vi "nanocal -- nuclear schottky fit V8.vi"() -> ()   [LabVIEW 2021] (continued)
\"στN\" -> 0.000000000000   ,  \"τ11 \" -> 0.000000000000   ,  \"τ12\" -> 0.000000000000   ,  \"τ22\" -> 0.000000000000   ,  \"τN1\" -> 0.000000000000   ,  \"τN2\" -> 0.000000000000   ,  \"σηlogτ1 \" -> 0.000000000000   ,  \"σηlogτS\" -> 0.000000000000   ,  \"σηlogτN\" -> 0.000000000000   ,  \"σlogτ1\" -> 0.000000000000   ,  \"σlogτS\" -> 0.000000000000   ,  \"σlogτN\" -> 0.000000000000   ,  \"σητ1\" -> 0.000000000000   ,  \"σητS \" -> 0.000000000000   ,  \"σητN\" -> 0.000000000000    |>   , \r\"IDS0217_210310_RAW_cal__ref_\" ->   <|    \"ζ\" -> 0.121305227705   ,  \"τ1\" -> 0.032098202143   ,  \"τS\" -> 0.011865067519   ,  \"τN\" -> 0.005878702730   ,  \"τC\" -> 0.002147559783   ,  \"κ0\" -> 0.000000001032   ,  \"mm1\" -> 0.000202614262   ,  \"mm2\" -> 0.011552455211   ,  \"mm3\" -> 0.042386874792   ,  \"T\" -> 0.197000000000   ,  \"B\" -> 0.000000000000   ,  \"θ\" -> 0.000000000000   ,  \"Reoff\" -> 0.000000000000   ,  \"Imoff\" -> 0.000000000000   ,  \"στ1\" -> 0.000000000000   ,  \"στS\" -> 0.000000000000   ,  \"στN\" -> 0.000000000000   ,  \"τ11 \" -> 0.000000000000   ,  \"τ12\" -> 0.000000000000   ,  \"τ22\" -> 0.000000000000   ,  \"τN1\" -> 0.000000000000   ,  \"τN2\" -> 0.000000000000   ,  \"σηlogτ1 \" -> 0.000000000000   ,  \"σηlogτS\" -> 0.000000000000   ,  \"σηlogτN\" -> 0.000000000000   ,  \"σlogτ1\" -> 0.000000000000   ,  \"σlogτS\" -> 0.000000000000   ,  \"σlogτN\" -> 0.000000000000   ,  \"σητ1\" -> 0.000000000000   ,  \"σητS \" -> 0.000000000000   ,  \"σητN\" -> 0.000000000000    |>   , \r\"IDS0217_210310_RAW_cal__sam_\" ->   <|    \"ζ\" -> 0.101804363109   ,  \"τ1\" -> 0.031947692776   ,  \"τS\" -> 0.014125667853   ,  \"τN\" -> 0.006009042128   ,  \"τC\" -> 0.002323789932   ,  \"κ0\" -> 0.000000001168   ,  \"mm1\" -> 0.000188754224   ,  \"mm2\" -> 0.013103876414   ,  \"mm3\" -> 0.043163363377   ,  \"T\" -> 0.197000000000   ,  \"B\" -> 0.000000000000   ,  \"θ\" -> 0.000000000000   ,  \"Reoff\" -> 0.000000000000   ,  \"Imoff\" -> 0.000000000000   ,  \"στ1\" -> 0.000000000000   ,  \"στS\" -> 0.000000000000   ,  \"στN\" -> 0.000000000000   ,  \"τ11 \" -> 0.000000000000   ,  \"τ12\" -> 0.000000000000   ,  \"τ22\" -> 0.000000000000   ,  \"τN1\" -> 0.000000000000   ,  \"τN2\" -> 0.000000000000   ,  \"σηlogτ1 \" -> 0.000000000000   ,  \"σηlogτS\" -> 0.000000000000   ,  \"σηlogτN\" -> 0.000000000000   ,  \"σlogτ1\" -> 0.000000000000   ,  \"σlogτS\" -> 0.000000000000   ,  \"σlogτN\" -> 0.000000000000   ,  \"σητ1\" -> 0.000000000000   ,  \"σητS \" -> 0.000000000000   ,  \"σητN\" -> 0.000000000000    |>   , \r\"IDS0218_210310_RAW_cal__ref_\" ->   <|    \"ζ\" -> 0.000000000000   ,  \"τ1\" -> 0.000000000000   ,  \"τS\" -> 0.000000000000   ,  \"τN\" -> 0.000000000000   ,  \"τC\" -> 0.000000000000   ,  \"κ0\" -> 0.000000000000   ,  \"mm1\" -> 0.000000000000   ,  \"mm2\" -> 0.000000000000   ,  \"mm3\" -> 0.000000000000   ,  \"T\" -> 1.550000000000   ,  \"B\" -> 0.000000000000   ,  \"θ\" -> 0.000000000000   ,  \"Reoff\" -> 0.000000000000   ,  \"Imoff\" -> 0.000000000000   ,  \"στ1\" -> 0.000000000000   ,  \"στS\" -> 0.000000000000   ,  \"στN\" -> 0.000000000000   ,  \"τ11 \" -> 0.000000000000   ,  \"τ12\" -> 0.000000000000   ,  \"τ22\" -> 0.000000000000   ,  \"τN1\" -> 0.000000000000   ,  \"τN2\" -> 0.000000000000   ,  \"σηlogτ1 \" -> 0.000000000000   ,  \"σηlogτS\" -> 0.000000000000   ,  \"σηlogτN\" -> 0.000000000000   ,  \"σlogτ1\" -> 0.000000000000   ,  \"σlogτS\" -> 0.000000000000   ,  \"σlogτN\" -> 0.000000000000   ,  \"σητ1\" -> 0.000000000000   ,  \"σητS \" -> 0.000000000000   ,  \"σητN\" -> 0.000000000000    |>   , \r\"IDS0218_210310_RAW_cal__sam_\" ->   <|    \"ζ\" -> 0.008537038929   ,  \"τ1\" -> 0.006154643814   ,  \"τS\" -> 0.040521205127   ,  \"τN\" -> 0.000711776675   ,  \"τC\" -> 0.001925410383   ,  \"κ0\" -> 0.000000011800   ,  \"mm1\" -> 0.000015570479   ,  \"mm2\" -> 0.006036709260   ,  \"mm3\" -> 0.043612763831   ,  \"T\" -> 1.550000000000   ,  \"B\" -> 0.000000000000   ,  \"θ\" -> 0.000000000000   ,  \"Reoff\" -> -420408.163265306153   ,  \"Imoff\" -> 0.000000000000   ,  \"στ1\" -> 0.000216261088   ,  \"στS\" -> 0.000541561495   ,  \"στN\" -> 0.000022390164   ,  \"τ11 \" -> 0.000000000000   ,  \"τ12\" -> 0.000000000000   ,  \"τ22\" -> 0.000000000000   ,  \"τN1\" -> 0.000000000000   ,  \"τN2\" -> 0.000000000000   ,  \"σηlogτ1 \" -> 0.000000000000   ,  \"σηlogτS\" -> 0.000000000000   ,  \"σηlogτN\" -> 0.000000000000   ,  \"σlogτ1\" -> 0.000000000000   ,  \"σlogτS\" -> 0.000000000000   ,  \"σlogτN\" -> 0.000000000000   ,  \"σητ1\" -> 0.000000000000   ,  \"σητS \" -> 0.000000000000   ,  \"σητN\" -> 0.000000000000    |>   , \r\"IDS0219_210310_RAW_cal__ref_\" ->   <|    \"ζ\" -> 0.000000000000   ,  \"τ1\" -> 0.000000000000   ,  \"τS\" -> 0.000000000000   ,  \"τN\" -> 0.000000000000   ,  \"τC\" -> 0.000000000000   ,  \"κ0\" -> 0.000000000000   ,  \"mm1\" -> 0.000000000000   ,  \"mm2\" -> 0.000000000000   ,  \"mm3\" -> 0.000000000000   ,  \"T\" -> 1.000000000000   ,  \"B\" -> 0.000000000000   ,  \"θ\" -> 0.000000000000   ,  \"Reoff\" -> 0.000000000000   ,  \"Imoff\" -> 0.000000000000   ,  \"στ1\" -> 0.000000000000   ,  \"στS\" -> 0.000000000000   ,  \"στN\" -> 0.000000000000   ,  \"τ11 \" -> 0.000000000000   ,  \"τ12\" -> 0.000000000000   ,  \"τ22\" -> 0.000000000000   ,  \"τN1\" -> 0.000000000000   ,  \"τN2\" -> 0.000000000000   ,  \"σηlogτ1 \" -> 0.000000000000   ,  \"σηlogτS\" -> 0.000000000000   ,  \"σηlogτN\" -> 0.000000000000   ,  \"σlogτ1\" -> 0.000000000000   ,  \"σlogτS\" -> 0.000000000000   ,  \"σlogτN\" -> 0.000000000000   ,  \"σητ1\" -> 0.000000000000   ,  \"σητS \" -> 0.000000000000   ,  \"σητN\" -> 0.000000000000    |>   , \r\"IDS0219_210310_RAW_cal__sam_\" ->   <|    \"ζ\" -> 0.000000000000   ,  \"τ1\" -> 0.000000000000   ,  \"τS\" -> 0.000000000000   ,  \"τN\" -> 0.000000000000   ,  \"τC\" -> 0.000000000000   ,  \"κ0\" -> 0.000000000000   ,  \"mm1\" -> 0.000000000000   ,  \"mm2\" -> 0.000000000000   ,  \"mm3\" -> 0.000000000000   ,  \"T\" -> 1.000000000000   ,  \"B\" -> 0.000000000000   ,  \"θ\" -> 0.000000000000   ,  \"Reoff\" -> 0.000000000000   ,  \"Imoff\" -> 0.000000000000   ,  \"στ1\" -> 0.000000000000   ,  \"στS\" -> 0.000000000000   ,  \"στN\" -> 0.000000000000   ,  \"τ11 \" -> 0.000000000000   ,  \"τ12\" -> 0.000000000000   ,  \"τ22\" -> 0.000000000000   ,  \"τN1\" -> 0.000000000000   ,  \"τN2\" -> 0.000000000000   ,  \"σηlogτ1 \" -> 0.000000000000   ,  \"σηlogτS\" -> 0.000000000000   ,  \"σηlogτN\" -> 0.000000000000   ,  \"σlogτ1\" -> 0.000000000000   ,  \"σlogτS\" -> 0.000000000000   ,  \"σlogτN\" -> 0.000000000000   ,  \"σητ1\" -> 0.000000000000   ,  \"σητS \" -> 0.000000000000   ,  \"σητN\" -> 0.000000000000    |>   , \r\"IDS0220_210310_RAW_cal__ref_\" ->   <|    \"ζ\" -> 0.000000000000   ,  \"τ1\" -> 0.000000000000   ,  \"τS\" -> 0.000000000000   ,  \"τN\" -> 0.000000000000   ,  \"τC\" -> 0.000000000000   ,  \"κ0\" -> 0.000000000000   ,  \"mm1\" -> 0.000000000000   ,  \"mm2\" -> 0.000000000000   ,  \"mm3\" -> 0.000000000000   ,  \"T\" -> 0.677000000000   ,  \"B\" -> 0.000000000000   ,  \"θ\" -> 0.000000000000   ,  \"Reoff\" -> 0.000000000000   ,  \"Imoff\" -> 0.000000000000   ,  \"στ1\" -> 0.000000000000   ,  \"στS\" -> 0.000000000000   ,  \"στN\" -> 0.000000000000   ,  \"τ11 \" -> 0.000000000000   ,  \"τ12\" -> 0.000000000000   ,  \"τ22\" -> 0.000000000000   ,  \"τN1\" -> 0.000000000000   ,  \"τN2\" -> 0.000000000000   ,  \"σηlogτ1 \" -> 0.000000000000   ,  \"σηlogτS\" -> 0.000000000000   ,  \"σηlogτN\" -> 0.000000000000   ,  \"σlogτ1\" -> 0.000000000000   ,  \"σlogτS\" -> 0.000000000000   ,  \"σlogτN\" -> 0.000000000000   ,  \"σητ1\" -> 0.000000000000   ,  \"σητS \" -> 0.000000000000   ,  \"σητN\" -> 0.000000000000    |>   , \r\"IDS0220_210310_RAW_cal__sam_\" ->   <|    \"ζ\" -> 0.000000000000   ,  \"τ1\" -> 0.000000000000   ,  \"τS\" -> 0.000000000000   ,  \"τN\" -> 0.000000000000   ,  \"τC\" -> 0.000000000000   ,  \"κ0\" -> 0.000000000000   ,  \"mm1\" -> 0.000000000000   ,  \"mm2\" -> 0.000000000000   ,  \"mm3\" -> 0.000000000000   ,  \"T\" -> 0.677000000000   ,  \"B\" -> 0.000000000000   ,  \"θ\" -> 0.000000000000   ,  \"Reoff\" -> 0.000000000000   ,  \"Imoff\" -> 0.000000000000   ,  \"στ1\" -> 0.000000000000   ,  \"στS\" -> 0.000000000000   ,  \"στN\" -> 0.000000000000   ,  \"τ11 \" -> 0.000000000000   ,  \"τ12\" -> 0.000000000000   ,  \"τ22\" -> 0.000000000000   ,  \"τN1\" -> 0.000000000000   ,  \"τN2\" -> 0.000000000000   ,  \"σηlogτ1 \" -> 0.000000000000   ,  \"σηlogτS\" -> 0.000000000000   ,  \"σηlogτN\" -> 0.000000000000   ,  \"σlogτ1\" -> 0.000000000000   ,  \"σlogτS\" -> 0.000000000000   ,  \"σlogτN\" -> 0.000000000000   ,  \"σητ1\" -> 0.000000000000   ,  \"σητS \" -> 0.000000000000   ,  \"σητN\" -> 0.000000000000    |>   , \r\"IDS0224_210310_RAW_cal__ref_\" ->   <|    \"ζ\" -> 0.000000000000   ,  \"τ1\" -> 0.000000000000   ,  \"τS\" -> 0.000000000000   ,  \"τN\" -> 0.000000000000   ,  \"τC\" -> 0.000000000000   ,  \"κ0\" -> 0.000000000000   ,  \"mm1\" -> 0.000000000000   ,  \"mm2\" -> 0.000000000000   ,  \"mm3\" -> 0.000000000000   ,  \"T\" -> 0.000000000000   ,  \"B\" -> 0.000000000000   ,  \"θ\" -> 0.000000000000   ,  \"Reoff\" -> 0.000000000000   ,  \"Imoff\" -> 0.000000000000   ,  \"στ1\" -> 0.000000000000   ,  \"στS\" -> 0.000000000000   ,  \"στN\" -> 0.000000000000   ,  \"τ11 \" -> 0.000000000000   ,  \"τ12\" -> 0.000000000000   ,  \"τ22\" -> 0.000000000000   ,  \"τN1\" -> 0.000000000000   ,  \"τN2\" -> 0.000000000000   ,  \"σηlogτ1 \" -> 0.000000000000   ,  \"σηlogτS\" -> 0.000000000000   ,  \"σηlogτN\" -> 0.000000000000   ,  \"σlogτ1\" -> 0.000000000000   ,  \"σlogτS\" -> 0.000000000000   ,  \"σlogτN\" -> 0.000000000000   ,  \"σητ1\" -> 0.000000000000   ,  \"σητS \" -> 0.000000000000   ,  \"σητN\" -> 0.000000000000    |>   , \r\"IDS0224_210310_RAW_cal__sam_\" ->   <|    \"ζ\" -> 0.000000000000   ,  \"τ1\" -> 0.000000000000   ,  \"τS\" -> 0.000000000000   ,  \"τN\" -> 0.000000000000   ,  \"τC\" -> 0.000000000000   ,  \"κ0\" -> 0.000000000000   ,  \"mm1\" -> 0.000000000000   ,  \"mm2\" -> 0.000000000000   ,  \"mm3\" -> 0.000000000000   ,  \"T\" -> 0.000000000000   ,  \"B\" -> 0.000000000000   ,  \"θ\" -> 0.000000000000   ,  \"Reoff\" -> 0.000000000000   ,  \"Imoff\" -> 0.000000000000   ,  \"στ1\" -> 0.000000000000   ,  \"στS\" -> 0.000000000000   ,  \"στN\" -> 0.000000000000   ,  \"τ11 \" -> 0.000000000000   ,  \"τ12\" -> 0.000000000000   ,  \"τ22\" -> 0.000000000000   ,  \"τN1\" -> 0.000000000000   ,  \"τN2\" -> 0.000000000000   ,  \"σηlogτ1 \" -> 0.000000000000   ,  \"σηlogτS\" -> 0.000000000000   ,  \"σηlogτN\" -> 0.000000000000   ,  \"σlogτ1\" -> 0.000000000000   ,  \"σlogτS\" -> 0.000000000000   ,  \"σlogτN\" -> 0.000000000000   ,  \"σητ1\" -> 0.000000000000   ,  \"σητS \" -> 0.000000000000   ,  \"σητN\" -> 0.000000000000    |>   , \r\"IDS0293_210427_RAW_cal__ref_\" ->   <|    \"ζ\" -> 0.016384838586   ,  \"τ1\" -> 0.013784349529   ,  \"τS\" -> 0.011495286759   ,  \"τN\" -> 0.000117117954   ,  \"τC\" -> 0.004048153799   ,  \"κ0\" -> 0.000000013122   ,  \"mm1\" -> 0.000048616206   ,  \"mm2\" -> 0.013163310838   ,  \"mm3\" -> 0.016423248374   ,  \"T\" -> 1.900000000000   ,  \"B\" -> 12.000000000000   ,  \"θ\" -> 30.000000000000   ,  \"Reoff\" -> 0.000000000000   ,  \"Imoff\" -> 0.000000000000   ,  \"στ1\" -> 0.000000000000   ,  \"στS\" -> 0.000000000000   ,  \"στN\" -> 0.000000000000   ,  \"τ11 \" -> 0.000000000000   ,  \"τ12\" -> 0.000000000000   ,  \"τ22\" -> 0.000000000000   ,  \"τN1\" -> 0.000000000000   ,  \"τN2\" -> 0.000000000000   ,  \"σηlogτ1 \" -> 0.000000000000   ,  \"σηlogτS\" -> 0.000000000000   ,  \"σηlogτN\" -> 0.000000000000   ,  \"σlogτ1\" -> 0.000000000000   ,  \"σlogτS\" -> 0.000000000000   ,  \"σlogτN\" -> 0.000000000000   ,  \"σητ1\" -> 0.000000000000   ,  \"σητS \" -> 0.000000000000   ,  \"σητN\" -> 0.000000000000    |>   , \r\"IDS0293_210427_RAW_cal__sam_\" ->   <|    \"ζ\" -> 0.009769235649   ,  \"τ1\" -> 0.020538276815   ,  \"τS\" -> 0.013494754544   ,  \"τN\" -> 0.000177075548   ,  \"τC\" -> 0.005872879859   ,  \"κ0\" -> 0.000000013933   ,  \"mm1\" -> 0.000039786676   ,  \"mm2\" -> 0.018120715591   ,  \"mm3\" -> 0.022056047829   ,  \"T\" -> 1.900000000000   ,  \"B\" -> 12.000000000000   ,  \"θ\" -> 30.000000000000   ,  \"Reoff\" -> -172000.000000000000   ,  \"Imoff\" -> 0.000000000000   ,  \"στ1\" -> 0.000000000000   ,  \"στS\" -> 0.000000000000   ,  \"στN\" -> 0.000000000000   ,  \"τ11 \" -> 0.000000000000   ,  \"τ12\" -> 0.000000000000   ,  \"τ22\" -> 0.000000000000   ,  \"τN1\" -> 0.000000000000   ,  \"τN2\" -> 0.000000000000   ,  \"σηlogτ1 \" -> 0.000000000000   ,  \"σηlogτS\" -> 0.000000000000   ,  \"σηlogτN\" -> 0.000000000000   ,  \"σlogτ1\" -> 0.000000000000   ,  \"σlogτS\" -> 0.000000000000   ,  \"σlogτN\" -> 0.000000000000   ,  \"σητ1\" -> 0.000000000000   ,  \"σητS \" -> 0.000000000000   ,  \"σητN\" -> 0.000000000000    |>   , \r\"IDS0294_210427_RAW_cal__ref_\" ->   <|    \"ζ\" -> 0.016199564893   ,  \"τ1\" -> 0.012483452644   ,  \"τS\" -> 0.017871115056   ,  \"τN\" -> 0.000512607924   ,  \"τC\" -> 0.002961380924   ,  \"κ0\" -> 0.000000007613   ,  \"mm1\" -> 0.000040667321   ,  \"mm2\" -> 0.011819109280   ,  \"mm3\" -> 0.022266588260   ,  \"T\" -> 1.130000000000   ,  \"B\" -> 12.000000000000   ,  \"θ\" -> 30.000000000000   ,  \"Reoff\" -> 0.000000000000   ,  \"Imoff\" -> 0.000000000000   ,  \"στ1\" -> 0.000093134340   ,  \"στS\" -> 0.000001485132   ,  \"στN\" -> 0.000001930575   ,  \"τ11 \" -> 0.000000000000   ,  \"τ12\" -> 0.000000000000   ,  \"τ22\" -> 0.000000000000   ,  \"τN1\" -> 0.000000000000   ,  \"τN2\" -> 0.000000000000   ,  \"σηlogτ1 \" -> 0.049343719847   ,  \"σηlogτS\" -> 0.000081625171   ,  \"σηlogτN\" -> 0.045732774165   ,  \"σlogτ1\" -> 0.007460623478   ,  \"σlogτS\" -> 0.000083102361   ,  \"σlogτN\" -> 0.003766182195   ,  \"σητ1\" -> 0.000615979990   ,  \"σητS \" -> 0.000001458733   ,  \"σητN\" -> 0.000023442982    |>   , \r\"IDS0294_210427_RAW_cal__sam_\" ->   <|    \"ζ\" -> 0.010952304636   ,  \"τ1\" -> 0.020329649306   ,  \"τS\" -> 0.020621176960   ,  \"τN\" -> 0.000487558003   ,  \"τC\" -> 0.005477732780   ,  \"κ0\" -> 0.000000008194   ,  \"mm1\" -> 0.000047079068   ,  \"mm2\" -> 0.019035053021   ,  \"mm3\" -> 0.028065174256   ,  \"T\" -> 1.130000000000   ,  \"B\" -> 12.000000000000   ,  \"θ\" -> 30.000000000000   ,  \"Reoff\" -> -250000.000000000000   ,  \"Imoff\" -> 0.000000000000   ,  \"στ1\" -> 0.000000000000   ,  \"στS\" -> 0.000000000000   ,  \"στN\" -> 0.000000000000   ,  \"τ11 \" -> 0.000000000000   ,  \"τ12\" -> 0.000000000000   ,  \"τ22\" -> 0.000000000000   ,  \"τN1\" -> 0.000000000000   ,  \"τN2\" -> 0.000000000000   ,  \"σηlogτ1 \" -> 0.000000000000   ,  \"σηlogτS\" -> 0.000000000000   ,  \"σηlogτN\" -> 0.000000000000   ,  \"σlogτ1\" -> 0.000000000000   ,  \"σlogτS\" -> 0.000000000000   ,  \"σlogτN\" -> 0.000000000000   ,  \"σητ1\" -> 0.000000000000   ,  \"σητS \" -> 0.000000000000   ,  \"σητN\" -> 0.000000000000    |>   , \r\"IDS0295_210427_RAW_cal__ref_\" ->   <|    \"ζ\" -> 0.020389261933   ,  \"τ1\" -> 0.010612152488   ,  \"τS\" -> 0.021498854544   ,  \"τN\" -> 0.000696262506   ,  \"τC\" -> 0.003673829836   ,  \"κ0\" -> 0.000000005447   ,  \"mm1\" -> 0.000063032876   ,  \"mm2\" -> 0.010144720198   ,  \"mm3\" -> 0.026725888355   ,  \"T\" -> 0.830000000000   ,  \"B\" -> 12.000000000000   ,  \"θ\" -> 30.000000000000   ,  \"Reoff\" -> 0.000000000000   ,  \"Imoff\" -> 0.000000000000   ,  \"στ1\" -> 0.000068445753   ,  \"στS\" -> 0.000002033603   ,  \"στN\" -> 0.000002213743   ,  \"τ11 \" -> 0.000000000000   ,  \"τ12\" -> 0.000000000000   ,  \"τ22\" -> 0.000000000000   ,  \"τN1\" -> 0.000000000000   ,  \"τN2\" -> 0.000000000000   ,  \"σηlogτ1 \" -> 0.060938855294   ,  \"σηlogτS\" -> 0.000153415303   ,  \"σηlogτN\" -> 0.047605279346   ,  \"σlogτ1\" -> 0.006449752127   ,  \"σlogτS\" -> 0.000094591209   ,  \"σlogτN\" -> 0.003179466662   ,  \"σητ1\" -> 0.000646692425   ,  \"σητS \" -> 0.000003298253   ,  \"σητN\" -> 0.000033145771    |>   , \r\"IDS0295_210427_RAW_cal__sam_\" ->   <|    \"ζ\" -> 0.014046811833   ,  \"τ1\" -> 0.021205417259   ,  \"τS\" -> 0.025982453768   ,  \"τN\" -> 0.000985536826   ,  \"τC\" -> 0.005692013080   ,  \"κ0\" -> 0.000000005890   ,  \"mm1\" -> 0.000064969808   ,  \"mm2\" -> 0.019619534974   ,  \"mm3\" -> 0.034559730440   ,  \"T\" -> 0.830000000000   ,  \"B\" -> 12.000000000000   ,  \"θ\" -> 30.000000000000   ,  \"Reoff\" -> -401999.999999999999   ,  \"Imoff\" -> 0.000000000000   ,  \"στ1\" -> 0.000000000000   ,  \"στS\" -> 0.000000000000   ,  \"στN\" -> 0.000000000000   ,  \"τ11 \" -> 0.000000000000   ,  \"τ12\" -> 0.000000000000   ,  \"τ22\" -> 0.000000000000   ,  \"τN1\" -> 0.000000000000   ,  \"τN2\" -> 0.000000000000   ,  \"σηlogτ1 \" -> 0.000000000000   ,  \"σηlogτS\" -> 0.000000000000   ,  \"σηlogτN\" -> 0.000000000000   ,  \"σlogτ1\" -> 0.000000000000   ,  \"σlogτS\" -> 0.000000000000   ,  \"σlogτN\" -> 0.000000000000   ,  \"σητ1\" -> 0.000000000000   ,  \"σητS \" -> 0.000000000000   ,  \"σητN\" -> 0.000000000000    |>   , \r\"IDS0296_210427_RAW_cal__ref_\" ->   <|    \"ζ\" -> 0.026639585484   ,  \"τ1\" -> 0.013378487833   ,  \"τS\" -> 0.026805002741   ,  \"τN\" -> 0.001646650498   ,  \"τC\" -> 0.002944101634   ,  \"κ0\" -> 0.000000003909   ,  \"mm1\" -> 0.000069166367   ,  \"mm2\" -> 0.012239451085   ,  \"mm3\" -> 0.033223565502   ,  \"T\" -> 0.620000000000   ,  \"B\" -> 12.000000000000   ,  \"θ\" -> 30.000000000000   ,  \"Reoff\" -> 0.000000000000   ,  \"Imoff\" -> 0.000000000000   ,  \"στ1\" -> 0.000041623267   ,  \"στS\" -> 0.000002241846   ,  \"στN\" -> 0.000002532014   ,  \"τ11 \" -> 0.000000000000   ,  \"τ12\" -> 0.000000000000   ,  \"τ22\" -> 0.000000000000   ,  \"τN1\" -> 0.000000000000   ,  \"τN2\" -> 0.000000000000   ,  \"σηlogτ1 \" -> 0.058801793000   ,  \"σηlogτS\" -> 0.000264248442   ,  \"σηlogτN\" -> 0.047506424516   ,  \"σlogτ1\" -> 0.003111208682   ,  \"σlogτS\" -> 0.000083635355   ,  \"σlogτN\" -> 0.001537675504   ,  \"σητ1\" -> 0.000786679072   ,  \"σητS \" -> 0.000007083180   ,  \"σητN\" -> 0.000078226478    |>   , \r\"IDS0296_210427_RAW_cal__sam_\" ->   <|    \"ζ\" -> 0.017388662959   ,  \"τ1\" -> 0.016835863979   ,  \"τS\" -> 0.033051741689   ,  \"τN\" -> 0.001876583642   ,  \"τC\" -> 0.004718731610   ,  \"κ0\" -> 0.000000004257   ,  \"mm1\" -> 0.000070854167   ,  \"mm2\" -> 0.015532685015   ,  \"mm3\" -> 0.041486738616   ,  \"T\" -> 0.620000000000   ,  \"B\" -> 12.000000000000   ,  \"θ\" -> 30.000000000000   ,  \"Reoff\" -> -602409.638554215430   ,  \"Imoff\" -> 0.000000000000   ,  \"στ1\" -> 0.000000000000   ,  \"στS\" -> 0.000000000000   ,  \"στN\" -> 0.000000000000   ,  \"τ11 \" -> 0.000000000000   ,  \"τ12\" -> 0.000000000000   ,  \"τ22\" -> 0.000000000000   ,  \"τN1\" -> 0.000000000000   ,  \"τN2\" -> 0.000000000000   ,  \"σηlogτ1 \" -> 0.000000000000   ,  \"σηlogτS\" -> 0.000000000000   ,  \"σηlogτN\" -> 0.000000000000   ,  \"σlogτ1\" -> 0.000000000000   ,  \"σlogτS\" -> 0.000000000000   ,  \"σlogτN\" -> 0.000000000000   ,  \"σητ1\" -> 0.000000000000   ,  \"σητS \" -> 0.000000000000   ,  \"σητN\" -> 0.000000000000    |>   , \r\"IDS0297_210427_RAW_cal__ref_\" ->   <|    \"ζ\" -> 0.032880006148   ,  \"τ1\" -> 0.011573992292   ,  \"τS\" -> 0.029546167136   ,  \"τN\" -> 0.002800651858   ,  \"τC\" -> 0.002501674064   ,  \"κ0\" -> 0.000000003300   ,  \"mm1\" -> 0.000073764511   ,  \"mm2\" -> 0.010265439642   ,  \"mm3\" -> 0.037146844804   ,  \"T\" -> 0.530000000000   ,  \"B\" -> 12.000000000000   ,  \"θ\" -> 30.000000000000   ,  \"Reoff\" -> 0.000000000000   ,  \"Imoff\" -> 0.000000000000   ,  \"στ1\" -> 0.000026464895   ,  \"στS\" -> 0.000003002676   ,  \"στN\" -> 0.000003189973   ,  \"τ11 \" -> 0.000000000000   ,  \"τ12\" -> 0.000000000000   ,  \"τ22\" -> 0.000000000000   ,  \"τN1\" -> 0.000000000000   ,  \"τN2\" -> 0.000000000000   ,  \"σηlogτ1 \" -> 0.067171330612   ,  \"σηlogτS\" -> 0.000538033954   ,  \"σηlogτN\" -> 0.049063862935   ,  \"σlogτ1\" -> 0.002286583119   ,  \"σlogτS\" -> 0.000101626575   ,  \"σlogτN\" -> 0.001139010991   ,  \"σητ1\" -> 0.000777440463   ,  \"σητS \" -> 0.000015896841   ,  \"σητN\" -> 0.000137410799    |>   , \r\"IDS0297_210427_RAW_cal__sam_\" ->   <|    \"ζ\" -> 0.020542184284   ,  \"τ1\" -> 0.020760439172   ,  \"τS\" -> 0.037341907366   ,  \"τN\" -> 0.003219016214   ,  \"τC\" -> 0.004292471555   ,  \"κ0\" -> 0.000000003557   ,  \"mm1\" -> 0.000077795275   ,  \"mm2\" -> 0.018267084885   ,  \"mm3\" -> 0.048102164115   ,  \"T\" -> 0.530000000000   ,  \"B\" -> 12.000000000000   ,  \"θ\" -> 30.000000000000   ,  \"Reoff\" -> -602409.638554215430   ,  \"Imoff\" -> 0.000000000000   ,  \"στ1\" -> 0.000000000000   ,  \"στS\" -> 0.000000000000   ,  \"στN\" -> 0.000000000000   ,  \"τ11 \" -> 0.000000000000   ,  \"τ12\" -> 0.000000000000   ,  \"τ22\" -> 0.000000000000   ,  \"τN1\" -> 0.000000000000   ,  \"τN2\" -> 0.000000000000   ,  \"σηlogτ1 \" -> 0.000000000000   ,  \"σηlogτS\" -> 0.000000000000   ,  \"σηlogτN\" -> 0.000000000000   ,  \"σlogτ1\" -> 0.000000000000   ,  \"σlogτS\" -> 0.000000000000   ,  \"σlogτN\" -> 0.000000000000   ,  \"σητ1\" -> 0.000000000000   ,  \"σητS \" -> 0.000000000000   ,  \"σητN\" -> 0.000000000000    |>   , \r\"IDS0298_210427_RAW_cal__ref_\" ->   <|    \"ζ\" -> 0.043729914910   ,  \"τ1\" -> 0.012982151341   ,  \"τS\" -> 0.033473880730   ,  \"τN\" -> 0.005072568857   ,  \"τC\" -> 0.001848506136   ,  \"κ0\" -> 0.000000002648   ,  \"mm1\" -> 0.000073701021   ,  \"mm2\" -> 0.010781606121   ,  \"mm3\" -> 0.044207432883   ,  \"T\" -> 0.430000000000   ,  \"B\" -> 12.000000000000   ,  \"θ\" -> 30.000000000000   ,  \"Reoff\" -> 0.000000000000   ,  \"Imoff\" -> 0.000000000000   ,  \"στ1\" -> 0.000015622195   ,  \"στS\" -> 0.000002788374   ,  \"στN\" -> 0.000003043175   ,  \"τ11 \" -> 0.000000000000   ,  \"τ12\" -> 0.000000000000   ,  \"τ22\" -> 0.000000000000   ,  \"τN1\" -> 0.000000000000   ,  \"τN2\" -> 0.000000000000   ,  \"σηlogτ1 \" -> 0.066709329762   ,  \"σηlogτS\" -> 0.000821711338   ,  \"σηlogτN\" -> 0.049548809037   ,  \"σlogτ1\" -> 0.001203359474   ,  \"σlogτS\" -> 0.000083299983   ,  \"σlogτN\" -> 0.000599927839   ,  \"σητ1\" -> 0.000866030615   ,  \"σητS \" -> 0.000027505867   ,  \"σητN\" -> 0.000251339746    |>   , \r\"IDS0298_210427_RAW_cal__sam_\" ->   <|    \"ζ\" -> 0.028504600675   ,  \"τ1\" -> 0.017787596977   ,  \"τS\" -> 0.043231501144   ,  \"τN\" -> 0.005920795525   ,  \"τC\" -> 0.002978583592   ,  \"κ0\" -> 0.000000002855   ,  \"mm1\" -> 0.000077491236   ,  \"mm2\" -> 0.014973532625   ,  \"mm3\" -> 0.056268519966   ,  \"T\" -> 0.430000000000   ,  \"B\" -> 12.000000000000   ,  \"θ\" -> 30.000000000000   ,  \"Reoff\" -> -2300000.000000000000   ,  \"Imoff\" -> 0.000000000000   ,  \"στ1\" -> 0.000000000000   ,  \"στS\" -> 0.000000000000   ,  \"στN\" -> 0.000000000000   ,  \"τ11 \" -> 0.000000000000   ,  \"τ12\" -> 0.000000000000   ,  \"τ22\" -> 0.000000000000   ,  \"τN1\" -> 0.000000000000   ,  \"τN2\" -> 0.000000000000   ,  \"σηlogτ1 \" -> 0.000000000000   ,  \"σηlogτS\" -> 0.000000000000   ,  \"σηlogτN\" -> 0.000000000000   ,  \"σlogτ1\" -> 0.000000000000   ,  \"σlogτS\" -> 0.000000000000   ,  \"σlogτN\" -> 0.000000000000   ,  \"σητ1\" -> 0.000000000000   ,  \"σητS \" -> 0.000000000000   ,  \"σητN\" -> 0.000000000000    |>   , \r\"IDS0299_210427_RAW_cal__ref_\" ->   <|    \"ζ\" -> 0.060514615834   ,  \"τ1\" -> 0.015692372838   ,  \"τS\" -> 0.037219144350   ,  \"τN\" -> 0.009623433713   ,  \"τC\" -> 0.001627271301   ,  \"κ0\" -> 0.000000002127   ,  \"mm1\" -> 0.000089367495   ,  \"mm2\" -> 0.011645867052   ,  \"mm3\" -> 0.055261648271   ,  \"T\" -> 0.360000000000   ,  \"B\" -> 12.000000000000   ,  \"θ\" -> 30.000000000000   ,  \"Reoff\" -> 0.000000000000   ,  \"Imoff\" -> 0.000000000000   ,  \"στ1\" -> 0.000012242681   ,  \"στS\" -> 0.000003204247   ,  \"στN\" -> 0.000003752483   ,  \"τ11 \" -> 0.000000000000   ,  \"τ12\" -> 0.000000000000   ,  \"τ22\" -> 0.000000000000   ,  \"τN1\" -> 0.000000000000   ,  \"τN2\" -> 0.000000000000   ,  \"σηlogτ1 \" -> 0.063518828231   ,  \"σηlogτS\" -> 0.001198828287   ,  \"σηlogτN\" -> 0.049895980082   ,  \"σlogτ1\" -> 0.000780167640   ,  \"σlogτS\" -> 0.000086091366   ,  \"σlogτN\" -> 0.000389931825   ,  \"σητ1\" -> 0.000996761135   ,  \"σητS \" -> 0.000044619363   ,  \"σητN\" -> 0.000480170657    |>   , \r\"IDS0299_210427_RAW_cal__sam_\" ->   <|    \"ζ\" -> 0.036443500348   ,  \"τ1\" -> 0.020154057220   ,  \"τS\" -> 0.048932682096   ,  \"τN\" -> 0.011280238135   ,  \"τC\" -> 0.002753749788   ,  \"κ0\" -> 0.000000002299   ,  \"mm1\" -> 0.000091994249   ,  \"mm2\" -> 0.015410264614   ,  \"mm3\" -> 0.069812837955   ,  \"T\" -> 0.360000000000   ,  \"B\" -> 12.000000000000   ,  \"θ\" -> 30.000000000000   ,  \"Reoff\" -> -2590361.445783123380   ,  \"Imoff\" -> 0.000000000000   ,  \"στ1\" -> 0.000000000000   ,  \"στS\" -> 0.000000000000   ,  \"στN\" -> 0.000000000000   ,  \"τ11 \" -> 0.000000000000   ,  \"τ12\" -> 0.000000000000   ,  \"τ22\" -> 0.000000000000   ,  \"τN1\" -> 0.000000000000   ,  \"τN2\" -> 0.000000000000   ,  \"σηlogτ1 \" -> 0.000000000000   ,  \"σηlogτS\" -> 0.000000000000   ,  \"σηlogτN\" -> 0.000000000000   ,  \"σlogτ1\" -> 0.000000000000   ,  \"σlogτS\" -> 0.000000000000   ,  \"σlogτN\" -> 0.000000000000   ,  \"σητ1\" -> 0.000000000000   ,  \"σητS \" -> 0.000000000000   ,  \"σητN\" -> 0.000000000000    |>   , \r\"IDS0300_210427_RAW_cal__ref_\" ->   <|    \"ζ\" -> 0.339239140566   ,  \"τ1\" -> 0.049004480747   ,  \"τS\" -> 0.154731734875   ,  \"τN\" -> 0.405076937535   ,  \"τC\" -> 0.001214632941   ,  \"κ0\" -> 0.000000000422   ,  \"mm1\" -> 0.000306310339   ,  \"mm2\" -> 0.012966272526   ,  \"mm3\" -> 0.786664216144   ,  \"T\" -> 0.140000000000   ,  \"B\" -> 12.000000000000   ,  \"θ\" -> 30.000000000000   ,  \"Reoff\" -> -103762048.192771077000   ,  \"Imoff\" -> 0.000000000000   ,  \"στ1\" -> 0.015510670555   ,  \"στS\" -> 0.015380063166   ,  \"στN\" -> 0.000000000000   ,  \"τ11 \" -> 0.000000000000   ,  \"τ12\" -> 0.000000000000   ,  \"τ22\" -> 0.000000000000   ,  \"τN1\" -> 0.000000000000   ,  \"τN2\" -> 0.000000000000   ,  \"σηlogτ1 \" -> 0.000000000000   ,  \"σηlogτS\" -> 0.000000000000   ,  \"σηlogτN\" -> 0.000000000000   ,  \"σlogτ1\" -> 0.000000000000   ,  \"σlogτS\" -> 0.000000000000   ,  \"σlogτN\" -> 0.000000000000   ,  \"σητ1\" -> 0.000000000000   ,  \"σητS \" -> 0.000000000000   ,  \"σητN\" -> 0.000000000000    |>   , \r\"IDS0300_210427_RAW_cal__sam_\" ->   <|    \"ζ\" -> 0.180438460866   ,  \"τ1\" -> 0.048255220427   ,  \"τS\" -> 0.195496614309   ,  \"τN\" -> 0.254134303670   ,  \"τC\" -> 0.001384159230   ,  \"κ0\" -> 0.000000000598   ,  \"mm1\" -> 0.000210501936   ,  \"mm2\" -> 0.019979803647   ,  \"mm3\" -> 0.560210702851   ,  \"T\" -> 0.140000000000   ,  \"B\" -> 12.000000000000   ,  \"θ\" -> 30.000000000000   ,  \"Reoff\" -> -29759036.144578307900   ,  \"Imoff\" -> 0.000000000000   ,  \"στ1\" -> 0.000000000000   ,  \"στS\" -> 0.000000000000   ,  \"στN\" -> 0.000000000000   ,  \"τ11 \" -> 0.000000000000   ,  \"τ12\" -> 0.000000000000   ,  \"τ22\" -> 0.000000000000   ,  \"τN1\" -> 0.000000000000   ,  \"τN2\" -> 0.000000000000   ,  \"σηlogτ1 \" -> 0.000000000000   ,  \"σηlogτS\" -> 0.000000000000   ,  \"σηlogτN\" -> 0.000000000000   ,  \"σlogτ1\" -> 0.000000000000   ,  \"σlogτS\" -> 0.000000000000   ,  \"σlogτN\" -> 0.000000000000   ,  \"σητ1\" -> 0.000000000000   ,  \"σητS \" -> 0.000000000000   ,  \"σητN\" -> 0.000000000000    |>   , \r\"IDS0301_210831_RAW_cal__ref_\" ->   <|    \"ζ\" -> 0.082126931999   ,  \"τ1\" -> 0.017305856709   ,  \"τS\" -> 0.041444693171   ,  \"τN\" -> 0.015130842560   ,  \"τC\" -> 0.001337765141   ,  \"κ0\" -> 0.000000001746   ,  \"mm1\" -> 0.000098793361   ,  \"mm2\" -> 0.011722113244   ,  \"mm3\" -> 0.068044626152   ,  \"T\" -> 0.300000000000   ,  \"B\" -> 12.000000000000   ,  \"θ\" -> 30.000000000000   ,  \"Reoff\" -> 0.000000000000   ,  \"Imoff\" -> 0.000000000000   ,  \"στ1\" -> 0.000019775099   ,  \"στS\" -> 0.000007122941   ,  \"στN\" -> 0.000008671110   ,  \"τ11 \" -> 0.000000000000   ,  \"τ12\" -> 0.000000000000   ,  \"τ22\" -> 0.000000000000   ,  \"τN1\" -> 0.000000000000   ,  \"τN2\" -> 0.000000000000   ,  \"σηlogτ1 \" -> 0.064027894608   ,  \"σηlogτS\" -> 0.001632596532   ,  \"σηlogτN\" -> 0.050896259041   ,  \"σlogτ1\" -> 0.001142682494   ,  \"σlogτS\" -> 0.000171866183   ,  \"σlogτN\" -> 0.000573075165   ,  \"σητ1\" -> 0.001108057569   ,  \"σητS \" -> 0.000067662462   ,  \"σητN\" -> 0.000770103282    |>   , \r\"IDS0301_210831_RAW_cal__sam_\" ->   <|    \"ζ\" -> 0.050368719514   ,  \"τ1\" -> 0.024372679774   ,  \"τS\" -> 0.056652990002   ,  \"τN\" -> 0.018868210601   ,  \"τC\" -> 0.002169557672   ,  \"κ0\" -> 0.000000001890   ,  \"mm1\" -> 0.000100537132   ,  \"mm2\" -> 0.016885854065   ,  \"mm3\" -> 0.088880953022   ,  \"T\" -> 0.300000000000   ,  \"B\" -> 12.000000000000   ,  \"θ\" -> 30.000000000000   ,  \"Reoff\" -> -5240963.855421677230   ,  \"Imoff\" -> 0.000000000000   ,  \"στ1\" -> 0.000000000000   ,  \"στS\" -> 0.000000000000   ,  \"στN\" -> 0.000000000000   ,  \"τ11 \" -> 0.000000000000   ,  \"τ12\" -> 0.000000000000   ,  \"τ22\" -> 0.000000000000   ,  \"τN1\" -> 0.000000000000   ,  \"τN2\" -> 0.000000000000   ,  \"σηlogτ1 \" -> 0.000000000000   ,  \"σηlogτS\" -> 0.000000000000   ,  \"σηlogτN\" -> 0.000000000000   ,  \"σlogτ1\" -> 0.000000000000   ,  \"σlogτS\" -> 0.000000000000   ,  \"σlogτN\" -> 0.000000000000   ,  \"σητ1\" -> 0.000000000000   ,  \"σητS \" -> 0.000000000000   ,  \"σητN\" -> 0.000000000000    |>   , \r\"IDS0302_210831_RAW_cal__ref_\" ->   <|    \"ζ\" -> 0.119117771190   ,  \"τ1\" -> 0.020484198431   ,  \"τS\" -> 0.046546118670   ,  \"τN\" -> 0.031746107320   ,  \"τC\" -> 0.001123547857   ,  \"κ0\" -> 0.000000001369   ,  \"mm1\" -> 0.000117314209   ,  \"mm2\" -> 0.011098056426   ,  \"mm3\" -> 0.098010597104   ,  \"T\" -> 0.250000000000   ,  \"B\" -> 12.000000000000   ,  \"θ\" -> 30.000000000000   ,  \"Reoff\" -> 0.000000000000   ,  \"Imoff\" -> 0.000000000000   ,  \"στ1\" -> 0.000013789764   ,  \"στS\" -> 0.000007768404   ,  \"στN\" -> 0.000010846329   ,  \"τ11 \" -> 0.000000000000   ,  \"τ12\" -> 0.000000000000   ,  \"τ22\" -> 0.000000000000   ,  \"τN1\" -> 0.000000000000   ,  \"τN2\" -> 0.000000000000   ,  \"σηlogτ1 \" -> 0.062827482470   ,  \"σηlogτS\" -> 0.002518670119   ,  \"σηlogτN\" -> 0.053009615785   ,  \"σlogτ1\" -> 0.000673190315   ,  \"σlogτS\" -> 0.000166896916   ,  \"σlogτN\" -> 0.000341658561   ,  \"σητ1\" -> 0.001286970618   ,  \"σητS \" -> 0.000117234318   ,  \"σητN\" -> 0.001682848952    |>   , \r\"IDS0302_210831_RAW_cal__sam_\" ->   <|    \"ζ\" -> 0.070275268573   ,  \"τ1\" -> 0.028026457127   ,  \"τS\" -> 0.065297867120   ,  \"τN\" -> 0.040008645873   ,  \"τC\" -> 0.001817885465   ,  \"κ0\" -> 0.000000001504   ,  \"mm1\" -> 0.000116520135   ,  \"mm2\" -> 0.015851021970   ,  \"mm3\" -> 0.126583756963   ,  \"T\" -> 0.250000000000   ,  \"B\" -> 12.000000000000   ,  \"θ\" -> 30.000000000000   ,  \"Reoff\" -> -8554216.867469877010   ,  \"Imoff\" -> 0.000000000000   ,  \"στ1\" -> 0.000000000000   ,  \"στS\" -> 0.000000000000   ,  \"στN\" -> 0.000000000000   ,  \"τ11 \" -> 0.000000000000   ,  \"τ12\" -> 0.000000000000   ,  \"τ22\" -> 0.000000000000   ,  \"τN1\" -> 0.000000000000   ,  \"τN2\" -> 0.000000000000   ,  \"σηlogτ1 \" -> 0.000000000000   ,  \"σηlogτS\" -> 0.000000000000   ,  \"σηlogτN\" -> 0.000000000000   ,  \"σlogτ1\" -> 0.000000000000   ,  \"σlogτS\" -> 0.000000000000   ,  \"σlogτN\" -> 0.000000000000   ,  \"σητ1\" -> 0.000000000000   ,  \"σητS \" -> 0.000000000000   ,  \"σητN\" -> 0.000000000000    |>   , \r\"IDS0303_210831_RAW_cal__ref_\" ->   <|    \"ζ\" -> 0.212927694685   ,  \"τ1\" -> 0.029784416053   ,  \"τS\" -> 0.063010370778   ,  \"τN\" -> 0.078316913737   ,  \"τC\" -> 0.000971683502   ,  \"κ0\" -> 0.000000001055   ,  \"mm1\" -> 0.000168791762   ,  \"mm2\" -> 0.012114302130   ,  \"mm3\" -> 0.189892783066   ,  \"T\" -> 0.200000000000   ,  \"B\" -> 12.000000000000   ,  \"θ\" -> 30.000000000000   ,  \"Reoff\" -> 0.000000000000   ,  \"Imoff\" -> 0.000000000000   ,  \"στ1\" -> 0.000061620932   ,  \"στS\" -> 0.000048874477   ,  \"στN\" -> 0.000083250584   ,  \"τ11 \" -> 0.000000000000   ,  \"τ12\" -> 0.000000000000   ,  \"τ22\" -> 0.000000000000   ,  \"τN1\" -> 0.000000000000   ,  \"τN2\" -> 0.000000000000   ,  \"σηlogτ1 \" -> 0.062829170044   ,  \"σηlogτS\" -> 0.003561984469   ,  \"σηlogτN\" -> 0.056674061290   ,  \"σlogτ1\" -> 0.002068898445   ,  \"σlogτS\" -> 0.000775657663   ,  \"σlogτN\" -> 0.001062996228   ,  \"σητ1\" -> 0.001871330141   ,  \"σητS \" -> 0.000224441962   ,  \"σητN\" -> 0.004438537569    |>   , \r\"IDS0303_210831_RAW_cal__sam_\" ->   <|    \"ζ\" -> 0.127771364483   ,  \"τ1\" -> 0.034431916362   ,  \"τS\" -> 0.086066228156   ,  \"τN\" -> 0.103317216156   ,  \"τC\" -> 0.001469970272   ,  \"κ0\" -> 0.000000001169   ,  \"mm1\" -> 0.000164317810   ,  \"mm2\" -> 0.014420189715   ,  \"mm3\" -> 0.234898604511   ,  \"T\" -> 0.200000000000   ,  \"B\" -> 12.000000000000   ,  \"θ\" -> 30.000000000000   ,  \"Reoff\" -> -17831325.301204815500   ,  \"Imoff\" -> 0.000000000000   ,  \"στ1\" -> 0.000000000000   ,  \"στS\" -> 0.000000000000   ,  \"στN\" -> 0.000000000000   ,  \"τ11 \" -> 0.000000000000   ,  \"τ12\" -> 0.000000000000   ,  \"τ22\" -> 0.000000000000   ,  \"τN1\" -> 0.000000000000   ,  \"τN2\" -> 0.000000000000   ,  \"σηlogτ1 \" -> 0.000000000000   ,  \"σηlogτS\" -> 0.000000000000   ,  \"σηlogτN\" -> 0.000000000000   ,  \"σlogτ1\" -> 0.000000000000   ,  \"σlogτS\" -> 0.000000000000   ,  \"σlogτN\" -> 0.000000000000   ,  \"σητ1\" -> 0.000000000000   ,  \"σητS \" -> 0.000000000000   ,  \"σητN\" -> 0.000000000000    |>   , \r\"IDS0304_210831_RAW_cal__ref_\" ->   <|    \"ζ\" -> 0.279635300057   ,  \"τ1\" -> 0.035679990389   ,  \"τS\" -> 0.085943482821   ,  \"τN\" -> 0.125379141268   ,  \"τC\" -> 0.000944269327   ,  \"κ0\" -> 0.000000000769   ,  \"mm1\" -> 0.000204959126   ,  \"mm2\" -> 0.013466168395   ,  \"mm3\" -> 0.293369021680   ,  \"T\" -> 0.170000000000   ,  \"B\" -> 12.000000000000   ,  \"θ\" -> 30.000000000000   ,  \"Reoff\" -> 0.000000000000   ,  \"Imoff\" -> 0.000000000000   ,  \"στ1\" -> 0.000147797307   ,  \"στS\" -> 0.000153583373   ,  \"στN\" -> 0.000257889382   ,  \"τ11 \" -> 0.000000000000   ,  \"τ12\" -> 0.000000000000   ,  \"τ22\" -> 0.000000000000   ,  \"τN1\" -> 0.000000000000   ,  \"τN2\" -> 0.000000000000   ,  \"σηlogτ1 \" -> 0.068151857614   ,  \"σηlogτS\" -> 0.004468282053   ,  \"σηlogτN\" -> 0.060259164916   ,  \"σlogτ1\" -> 0.004142302323   ,  \"σlogτS\" -> 0.001787027566   ,  \"σlogτN\" -> 0.002056876282   ,  \"σητ1\" -> 0.002431657625   ,  \"σητS \" -> 0.000384019722   ,  \"σητN\" -> 0.007555242351    |>   , \r\"IDS0304_210831_RAW_cal__sam_\" ->   <|    \"ζ\" -> 0.166070461716   ,  \"τ1\" -> 0.041003941798   ,  \"τS\" -> 0.114733330952   ,  \"τN\" -> 0.164402286708   ,  \"τC\" -> 0.001371627013   ,  \"κ0\" -> 0.000000000890   ,  \"mm1\" -> 0.000193629021   ,  \"mm2\" -> 0.015725118152   ,  \"mm3\" -> 0.351948620204   ,  \"T\" -> 0.170000000000   ,  \"B\" -> 12.000000000000   ,  \"θ\" -> 30.000000000000   ,  \"Reoff\" -> -32409638.554216861700   ,  \"Imoff\" -> 0.000000000000   ,  \"στ1\" -> 0.000000000000   ,  \"στS\" -> 0.000000000000   ,  \"στN\" -> 0.000000000000   ,  \"τ11 \" -> 0.000000000000   ,  \"τ12\" -> 0.000000000000   ,  \"τ22\" -> 0.000000000000   ,  \"τN1\" -> 0.000000000000   ,  \"τN2\" -> 0.000000000000   ,  \"σηlogτ1 \" -> 0.000000000000   ,  \"σηlogτS\" -> 0.000000000000   ,  \"σηlogτN\" -> 0.000000000000   ,  \"σlogτ1\" -> 0.000000000000   ,  \"σlogτS\" -> 0.000000000000   ,  \"σlogτN\" -> 0.000000000000   ,  \"σητ1\" -> 0.000000000000   ,  \"σητS \" -> 0.000000000000   ,  \"σητN\" -> 0.000000000000    |>   , \r\"IDS0305_210831_RAW_cal__ref_\" ->   <|    \"ζ\" -> 0.290525285970   ,  \"τ1\" -> 0.037812852216   ,  \"τS\" -> 0.093512516814   ,  \"τN\" -> 0.167160206336   ,  \"τC\" -> 0.000940281173   ,  \"κ0\" -> 0.000000000650   ,  \"mm1\" -> 0.000210392391   ,  \"mm2\" -> 0.012673110473   ,  \"mm3\" -> 0.362274371113   ,  \"T\" -> 0.160000000000   ,  \"B\" -> 12.000000000000   ,  \"θ\" -> 30.000000000000   ,  \"Reoff\" -> 0.000000000000   ,  \"Imoff\" -> 0.000000000000   ,  \"στ1\" -> 0.000149061244   ,  \"στS\" -> 0.000178639868   ,  \"στN\" -> 0.000324327167   ,  \"τ11 \" -> 0.000000000000   ,  \"τ12\" -> 0.000000000000   ,  \"τ22\" -> 0.000000000000   ,  \"τN1\" -> 0.000000000000   ,  \"τN2\" -> 0.000000000000   ,  \"σηlogτ1 \" -> 0.068993027609   ,  \"σηlogτS\" -> 0.004892524853   ,  \"σηlogτN\" -> 0.062584298965   ,  \"σlogτ1\" -> 0.003942078813   ,  \"σlogτS\" -> 0.001910331087   ,  \"σlogτN\" -> 0.001940217555   ,  \"σητ1\" -> 0.002608823157   ,  \"σητS \" -> 0.000457512313   ,  \"σητN\" -> 0.010461604328    |>   , \r\"IDS0305_210831_RAW_cal__sam_\" ->   <|    \"ζ\" -> 0.168984978681   ,  \"τ1\" -> 0.042944879888   ,  \"τS\" -> 0.137797235983   ,  \"τN\" -> 0.201278537585   ,  \"τC\" -> 0.001423239236   ,  \"κ0\" -> 0.000000000771   ,  \"mm1\" -> 0.000204183123   ,  \"mm2\" -> 0.016435652766   ,  \"mm3\" -> 0.424102769171   ,  \"T\" -> 0.160000000000   ,  \"B\" -> 12.000000000000   ,  \"θ\" -> 30.000000000000   ,  \"Reoff\" -> -36385542.168674692500   ,  \"Imoff\" -> 0.000000000000   ,  \"στ1\" -> 0.000000000000   ,  \"στS\" -> 0.000000000000   ,  \"στN\" -> 0.000000000000   ,  \"τ11 \" -> 0.000000000000   ,  \"τ12\" -> 0.000000000000   ,  \"τ22\" -> 0.000000000000   ,  \"τN1\" -> 0.000000000000   ,  \"τN2\" -> 0.000000000000   ,  \"σηlogτ1 \" -> 0.000000000000   ,  \"σηlogτS\" -> 0.000000000000   ,  \"σηlogτN\" -> 0.000000000000   ,  \"σlogτ1\" -> 0.000000000000   ,  \"σlogτS\" -> 0.000000000000   ,  \"σlogτN\" -> 0.000000000000   ,  \"σητ1\" -> 0.000000000000   ,  \"σητS \" -> 0.000000000000   ,  \"σητN\" -> 0.000000000000    |>   , \r\"IDS0306_210831_RAW_cal__ref_\" ->   <|    \"ζ\" -> 0.013593052641   ,  \"τ1\" -> 0.010989385662   ,  \"τS\" -> 0.007947176041   ,  \"τN\" -> 0.000037757079   ,  \"τC\" -> 0.003572854733   ,  \"κ0\" -> 0.000000023548   ,  \"mm1\" -> 0.000033287498   ,  \"mm2\" -> 0.010587625602   ,  \"mm3\" -> 0.012034800032   ,  \"T\" -> 3.100000000000   ,  \"B\" -> 12.000000000000   ,  \"θ\" -> 30.000000000000   ,  \"Reoff\" -> 0.000000000000   ,  \"Imoff\" -> 0.000000000000   ,  \"στ1\" -> 0.000000000000   ,  \"στS\" -> 0.000000000000   ,  \"στN\" -> 0.000000000000   ,  \"τ11 \" -> 0.000000000000   ,  \"τ12\" -> 0.000000000000   ,  \"τ22\" -> 0.000000000000   ,  \"τN1\" -> 0.000000000000   ,  \"τN2\" -> 0.000000000000   ,  \"σηlogτ1 \" -> 0.000000000000   ,  \"σηlogτS\" -> 0.000000000000   ,  \"σηlogτN\" -> 0.000000000000   ,  \"σlogτ1\" -> 0.000000000000   ,  \"σlogτS\" -> 0.000000000000   ,  \"σlogτN\" -> 0.000000000000   ,  \"σητ1\" -> 0.000000000000   ,  \"σητS \" -> 0.000000000000   ,  \"σητN\" -> 0.000000000000    |>   , \r\"IDS0306_210831_RAW_cal__sam_\" ->   <|    \"ζ\" -> 0.007685785961   ,  \"τ1\" -> 0.018036205476   ,  \"τS\" -> 0.008821186550   ,  \"τN\" -> 0.000090733660   ,  \"τC\" -> 0.005794291982   ,  \"κ0\" -> 0.000000024405   ,  \"mm1\" -> 0.000026803010   ,  \"mm2\" -> 0.014306219949   ,  \"mm3\" -> 0.018477889820   ,  \"T\" -> 3.100000000000   ,  \"B\" -> 12.000000000000   ,  \"θ\" -> 30.000000000000   ,  \"Reoff\" -> -62000.000000000000   ,  \"Imoff\" -> 0.000000000000   ,  \"στ1\" -> 0.000000000000   ,  \"στS\" -> 0.000000000000   ,  \"στN\" -> 0.000000000000   ,  \"τ11 \" -> 0.000000000000   ,  \"τ12\" -> 0.000000000000   ,  \"τ22\" -> 0.000000000000   ,  \"τN1\" -> 0.000000000000   ,  \"τN2\" -> 0.000000000000   ,  \"σηlogτ1 \" -> 0.000000000000   ,  \"σηlogτS\" -> 0.000000000000   ,  \"σηlogτN\" -> 0.000000000000   ,  \"σlogτ1\" -> 0.000000000000   ,  \"σlogτS\" -> 0.000000000000   ,  \"σlogτN\" -> 0.000000000000   ,  \"σητ1\" -> 0.000000000000   ,  \"σητS \" -> 0.000000000000   ,  \"σητN\" -> 0.000000000000    |>   , \r\"IDS0310_210901_RAW_cal__ref_\" ->   <|    \"ζ\" -> 0.303797102246   ,  \"τ1\" -> 0.049153401602   ,  \"τS\" -> 0.056270040032   ,  \"τN\" -> 0.227060279898   ,  \"τC\" -> 0.000912794118 
